vi "2 Tap 16-Bit.vi"() -> (0 "Pixels":cluster{"Pixel 0":u16, "Pixel 1":u16})   [LabVIEW 2015]
uses:
  <vilib>/rvi/eio/common/nirviEmuTemplateMethod_errors.vi
  <vilib>/eio/EIONode/EIONode.xnode
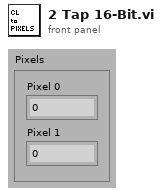
[diagram p1: front panel]
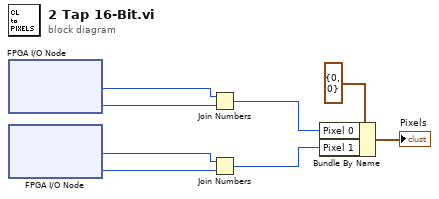
[diagram p0: block diagram]
diagram:
  n1 = xnode "FPGA I/O Node"() -> ("CL Port B"=w2:u8, "CL Port A"=w6:u8)  [unwired: 2 in, 2 out]
  n2 = xnode "FPGA I/O Node"() -> ("CL Port E"=w1:u8, "CL Port D"=w5:u8)  [unwired: 2 in, 2 out]
  n3 = Join Numbers(hi=w2, lo=w6) -> ((hi.lo)=w4:u16)
  n4 = Join Numbers(hi=w1, lo=w5) -> ((hi.lo)=w3:u16)
  n5 = Bundle By Name(cluster=cluster{"Pixel 0":u16, "Pixel 1":u16} {"Pixel 0"=0, "Pixel 1"=0} ("PixelData"), "Pixel 0"=w4, "Pixel 1"=w3) -> (→"Pixels":cluster{"Pixel 0":u16, "Pixel 1":u16})
